vi "Test Case Test Time Reset on Test Start.vi"(8 "error in (no error)":errorcluster, 11 "Result Model Result Recording Test in":refnum<class "Result Model Result Recording Test.lvclass">) -> (0 "error out":errorcluster, 3 "Result Model Result Recording Test out":refnum<class "Result Model Result Recording Test.lvclass">)   [LabVIEW 2020, in "Result Model Result Recording Test.lvclass"]
uses:
  Result Model Result Recording Test.lvclass
  source/Core/Result/Type.ctl
  source/Core/Result/Result.lvlib
  source/Core/Result/Status.ctl
  source/Core/Result/Result.ctl
  ae2c71b8-32bb-49d1-8500-0119bfec74ff.vi
  source/User Interface/Result Model/Result Model.lvclass
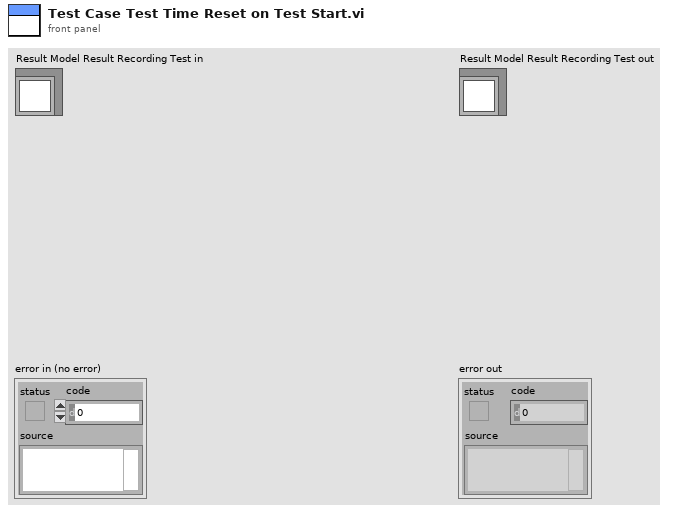
[diagram p1: front panel]
types:
  T1 = typedef "Result.lvlib/Result.ctl" = cluster{"Name":string, "Description":string, "Status":T2, "Result Type":T3, "Execution Time":dbl, "Data":cluster{"Expected":variant, "Actual":variant, "Delta":variant}}
  T2 = typedef "Result.lvlib/Status.ctl" = enum16{"", "Passed", "Failed", "Error", "Skipped", "Setup Error", "Broken", "Teardown Error"}
  T3 = typedef "Result.lvlib/Type.ctl" = enum16{"Test Case", "Test Suite", "Test Run", "Pass", "Fail", "Skip", "Pass if", "Fail if", "Pass if Error", "Fail if Error", "Pass if Equal", "Fail if Equal"}
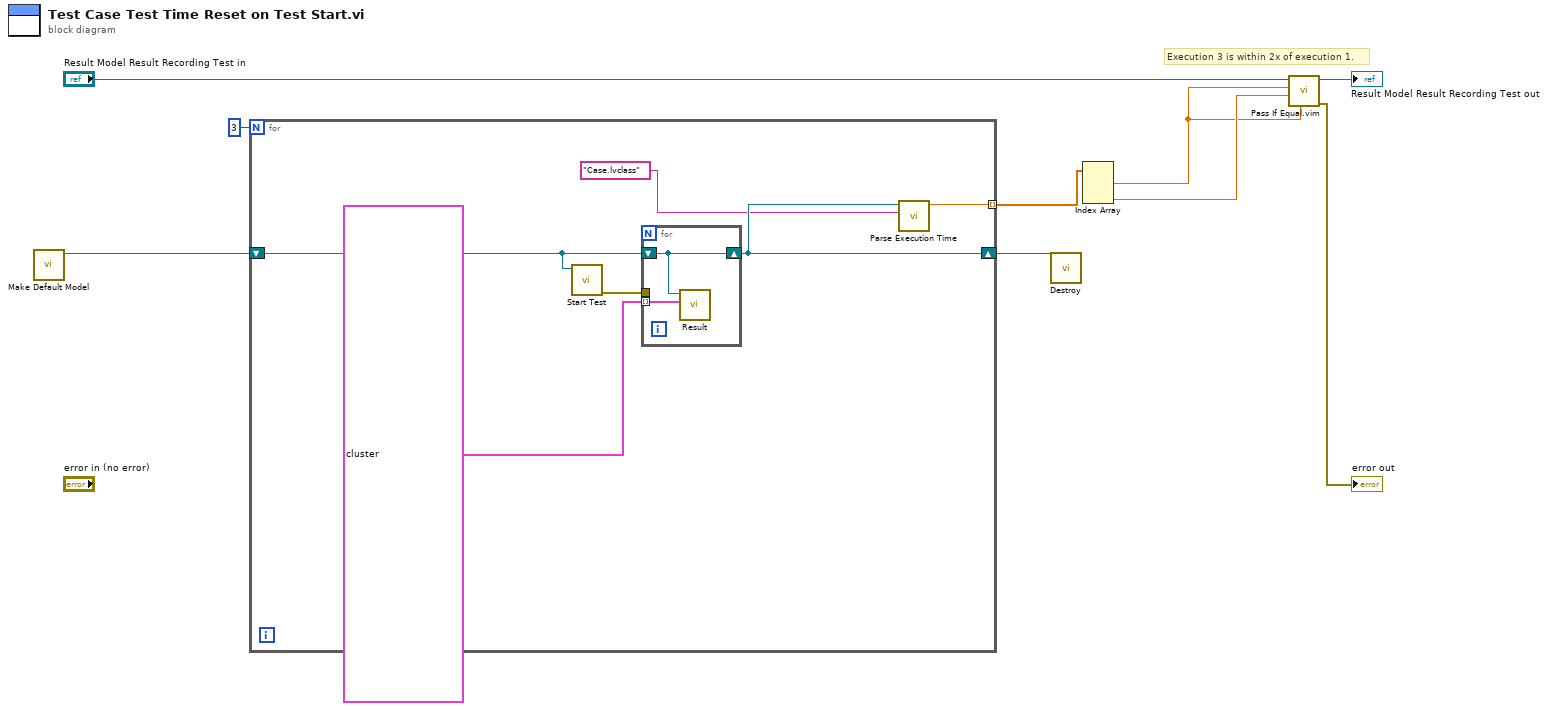
[diagram p0: block diagram]
diagram:
  # "Execution 3 is within 2x of execution 1."
  n1 = call "Make Default Model.vi"() -> ("Result Model out"=w9:refnum<class "Result Model.lvclass">)  [unwired: 10 in, 1 out]
  n2 = for {
    N: 3 -> [_]
    shift-right: [w14] -> w4
    shift-left: w9 -> [w11]
    tunnel: [w12] -> w1 mode=indexing
    n3 = call "Start Test.vi"("Result Model by Reference In"=w11) -> ("error out"=w10:errorcluster)  [unwired: 10 in]
    n4 = for {
      tunnel: T1[] [{"Name"="Case.lvclass:Test Method.vi", "Description"="Failed:\nMessage", "Status"=enum."Failed", "Result Type"=enum."Pass", "Execution Time"=0.0, "Data"={"Expected"=variant, "Actual"=variant, "Delta"=variant}}, {"Name"="Case.lvclass:Test Method.vi", "Description"="", "Status"=enum."Passed", "Result Type"=enum."Test Case", "Execution Time"=0.107, "Data"={"Expected"=variant, "Actual"=variant, "Delta"=variant}}] ("Results") -> [w17] mode=indexing
      shift-right: [w16] -> w14
      shift-left: w11 -> [w16]
      tunnel: w10 -> [_]
      n5 = call-dynamic "Result.vi"("Results"=w17, "Result Model by Reference In"=w16) -> ()  [unwired: 9 in, 1 out]
    }
    n6 = call "Parse Execution Time.vi"("Item"="Case.lvclass", "Result Model in"=w14) -> ("Numeric"=w12:dbl)  [unwired: 9 in]
  }
  n7 = call "Destroy.vi"("Result Model in"=w4) -> ()  [unwired: 10 in, 1 out]
  n8 = Index Array(array=w1) -> (element #1=w2:dbl, element #3=w3:dbl)  [unwired: 3 in, 1 out]
  n9 = call "Pass If Equal.vim"("Delta"=w2, "Actual"=w3, "Expected"=w2, "LUnit Test Case In"="Result Model Result Recording Test in") -> ("error out"=→"error out":errorcluster, "LUnit Test Case Out"=→"Result Model Result Recording Test out":refnum<class "Result Model Result Recording Test.lvclass">)  [unwired: 6 in]
